vi "IV_Reader.vi"(6 "Sweep parameters":T1={"Vbg"=15.0, "Vbg step"=0.0, "Vsg"=-0.5, "Vsg step"=0.025, "B"=0.0, "B step"=0.0, "Temp"=2.0, "Temp step"=0.0}, 7 "Path to PNG Folder":path=path "C:/Users/ansom/Desktop/Agilent/PNG's From Graphs/B_BG_7to-7", 8 "Use only a subset of the folder":bool, 9 "Subset Length":i32=41, 10 "Subset Index":i32=2624, 11 "Folder or File":path=path "D:/SA03008H.20180718/77_B+SG_B_-7to0inc1_SG_-0.5to0.5inc0.25_at0.2Hz_-300mVto-100mV_IV_@BG15") -> (3 "dIdV_Intensity_Output":dbl[][](array[numeric]))   [LabVIEW 2016]
uses:
  <userlib>/LevyLab/LV to ITX/LVtoITX.lvclass
  <vilib>/Analysis/NI_AALBase.lvlib
  <vilib>/MakerHub/Toolbox/LMH-Toolbox.lvlib
  <vilib>/Analysis/1siggen.llb/Ramp Pattern by Delta.vi
panel:
  out "initialized array":dbl[](array[numeric])
  out "output array":dbl[](array[numeric])
  out "output cluster":cluster{dbl[], dbl[], dbl[]}
  in  "Sgstep":dbl
  in  "Sgstart":dbl
  in  "T-Slider, F-AutoChopper":bool
  in  "dI/dV OFFSET":dbl=100.0 format="%#_13g"
  in  "IV OFFSET":dbl format="%#_13g"
  in  "e^2/h ?":bool
  in  "X step":dbl
  in  "X start":dbl
  out "Differential Conductance":dbl[][](graph)
  in  "Portion of data":cluster{dbl, dbl}(slide)={1.0, 0.0} scale=0.0..1.0
  out "Iterations of loop":i32=40
  out "directory":bool=TRUE
  out "dI/dV":cluster{dbl[], dbl[]}[](graph)
  out "A vs B":cluster{dbl[], dbl[]}[](graph)
  in  "Diff bin size":dbl
  out "Comments":string="IGOR\nX// Date: 7/19/2018 8:23 PM\nX// SA03008H\nX// \nX// Trying to see what the stepping stuff looks like up close\nX// \nX// Source 2 Drain 28 (lockin 1 and 7)\nX// Gohm resistor, sweep SG\nX// \nX// 100mV AC -200mV DC for the IV sweep\nX// \nX// -0.5 to 0.5 @ 0.025 V step sizes\nX// B at 4T now\n\nX// DSA_Vsg1=0.500000\n\nX// \nX// B= 3.999994\n\n\n\n\n\n\n\n\n\n\n\n\n\n\n\n\n\n\n\n\n\n\n\n\n\n\n\n\n\n\n\n\n\n\n\n\n\n\n\n\nX \nX Display/R 'time.SA03008H.20180718.000040'\nX AppendToGraph 'temp.SA03008H.20180718.000040'\nX AppendToGraph 'B.SA03008H.20180718.000040'\nX AppendToGraph 'Vsource.SA03008H.20180718.000040'\nX AppendToGraph 'Lockin0.SA03008H.20180718.000040'\nX AppendToGraph 'Lockin1.SA03008H.20180718.000040'\nX AppendToGraph 'Lockin2.SA03008H.20180718.000040'\nX AppendToGraph 'Lockin3.SA03008H.20180718.000040'\nX AppendToGraph 'Lockin4.SA03008H.20180718.000040'\nX AppendToGraph 'Lockin5.SA03008H.20180718.000040'\nX AppendToGraph 'B_rate.SA03008H.20180718.000040'\nX AppendToGraph 'DC0.SA03008H.20180718.000040'\nX AppendToGraph 'DC1.SA03008H.20180718.000040'\nX AppendToGraph 'DC2.SA03008H.20180718.000040'\nX AppendToGraph 'DC3.SA03008H.20180718.000040'\nX AppendToGraph 'DC4.SA03008H.20180718.000040'\nX AppendToGraph 'DC5.SA03008H.20180718.000040'\nX AppendToGraph 'DC6.SA03008H.20180718.000040'\nX AppendToGraph 'DC7.SA03008H.20180718.000040'\nX Label bottom \"x label\"\nX Label left \"y label\"\nX ModifyGraph rgb('time.SA03008H.20180718.000040')=(65280,0,0)\nX ModifyGraph rgb('temp.SA03008H.20180718.000040')=(65280,18432,0)\nX ModifyGraph rgb('B.SA03008H.20180718.000040')=(65280,36864,0)\nX ModifyGraph rgb('Vsource.SA03008H.20180718.000040')=(65280,55296,0)\nX ModifyGraph rgb('Lockin0.SA03008H.20180718.000040')=(57344,65280,0)\nX ModifyGraph rgb('Lockin1.SA03008H.20180718.000040')=(37376,65280,0)\nX ModifyGraph rgb('Lockin2.SA03008H.20180718.000040')=(18944,65280,0)\nX ModifyGraph rgb('Lockin3.SA03008H.20180718.000040')=(512,65280,0)\nX ModifyGraph rgb('Lockin4.SA03008H.20180718.000040')=(0,65280,17920)\nX ModifyGraph rgb('Lockin5.SA03008H.20180718.000040')=(0,65280,36352)\nX ModifyGraph rgb('B_rate.SA03008H.20180718.000040')=(0,65280,54784)\nX ModifyGraph rgb('DC0.SA03008H.20180718.000040')=(0,57856,65280)\nX ModifyGraph rgb('DC1.SA03008H.20180718.000040')=(0,39424,65280)\nX ModifyGraph rgb('DC2.SA03008H.20180718.000040')=(0,20992,65280)\nX ModifyGraph rgb('DC3.SA03008H.20180718.000040')=(0,2560,65280)\nX ModifyGraph rgb('DC4.SA03008H.20180718.000040')=(17408,0,65280)\nX ModifyGraph rgb('DC5.SA03008H.20180718.000040')=(35840,0,65280)\nX ModifyGraph rgb('DC6.SA03008H.20180718.000040')=(54272,0,65280)\nX ModifyGraph rgb('DC7.SA03008H.20180718.000040')=(65280,0,58368)\nX Legend/C/N=text0/J \"\\\\s('time.SA03008H.20180718.000040') time\\r\\\\s('temp.SA03008H.20180718.000040') temp\\r\\\\s('B.SA03008H.20180718.000040') B\\r\\\\s('Vsource.SA03008H.20180718.000040') Vsource\\r\\\\s('Lockin0.SA03008H.20180718.000040') Lockin0\\r\\\\s('Lockin1.SA03008H.20180718.000040') Lockin1\\r\\\\s('Lockin2.SA03008H.20180718.000040') Lockin2\\r\\\\s('Lockin3.SA03008H.20180718.000040') Lockin3\\r\\\\s('Lockin4.SA03008H.20180718.000040') Lockin4\\r\\\\s('Lockin5.SA03008H.20180718.000040') Lockin5\\r\\\\s('B_rate.SA03008H.20180718.000040') B_rate\\r\\\\s('DC0.SA03008H.20180718.000040') DC0\\r\\\\s('DC1.SA03008H.20180718.000040') DC1\\r\\\\s('DC2.SA03008H.20180718.000040') DC2\\r\\\\s('DC3.SA03008H.20180718.000040') DC3\\r\\\\s('DC4.SA03008H.20180718.000040') DC4\\r\\\\s('DC5.SA03008H.20180718.000040') DC5\\r\\\\s('DC6.SA03008H.20180718.000040') DC6\\r\\\\s('DC7.SA03008H.20180718.000040') DC7\"\nX ModifyGraph mirror(bottom)=1\nX ModifyGraph width=216\nX ModifyGraph height={Aspect,0.6}\nX ModifyGraph Log(bottom)=0\nX ModifyGraph Log(left)=0\nX \n"
  in  "Diff bin size":dbl=2.0
  out "N__":cluster{"N1":dbl, "N2":dbl, "N3":dbl, "N4":dbl}={"N1"=3614891004.465372, "N2"=3614891004.465372, "N3"=3614891004.465372, "N4"=3614891004.465372} {"N4" format="%#_6p"; "N3" format="%#_6p"; "N2" format="%#_6p"; "N1" format="%#_6p"}
  out "IV":dbl[][](graph)
  in  "index":T2={"A"=5, "B"=3, "C"=2, "D"=0, "E"=3, "N1"=0, "N2"=0, "N3"=0, "N4"=0}
  # "YES"
  # "NO"
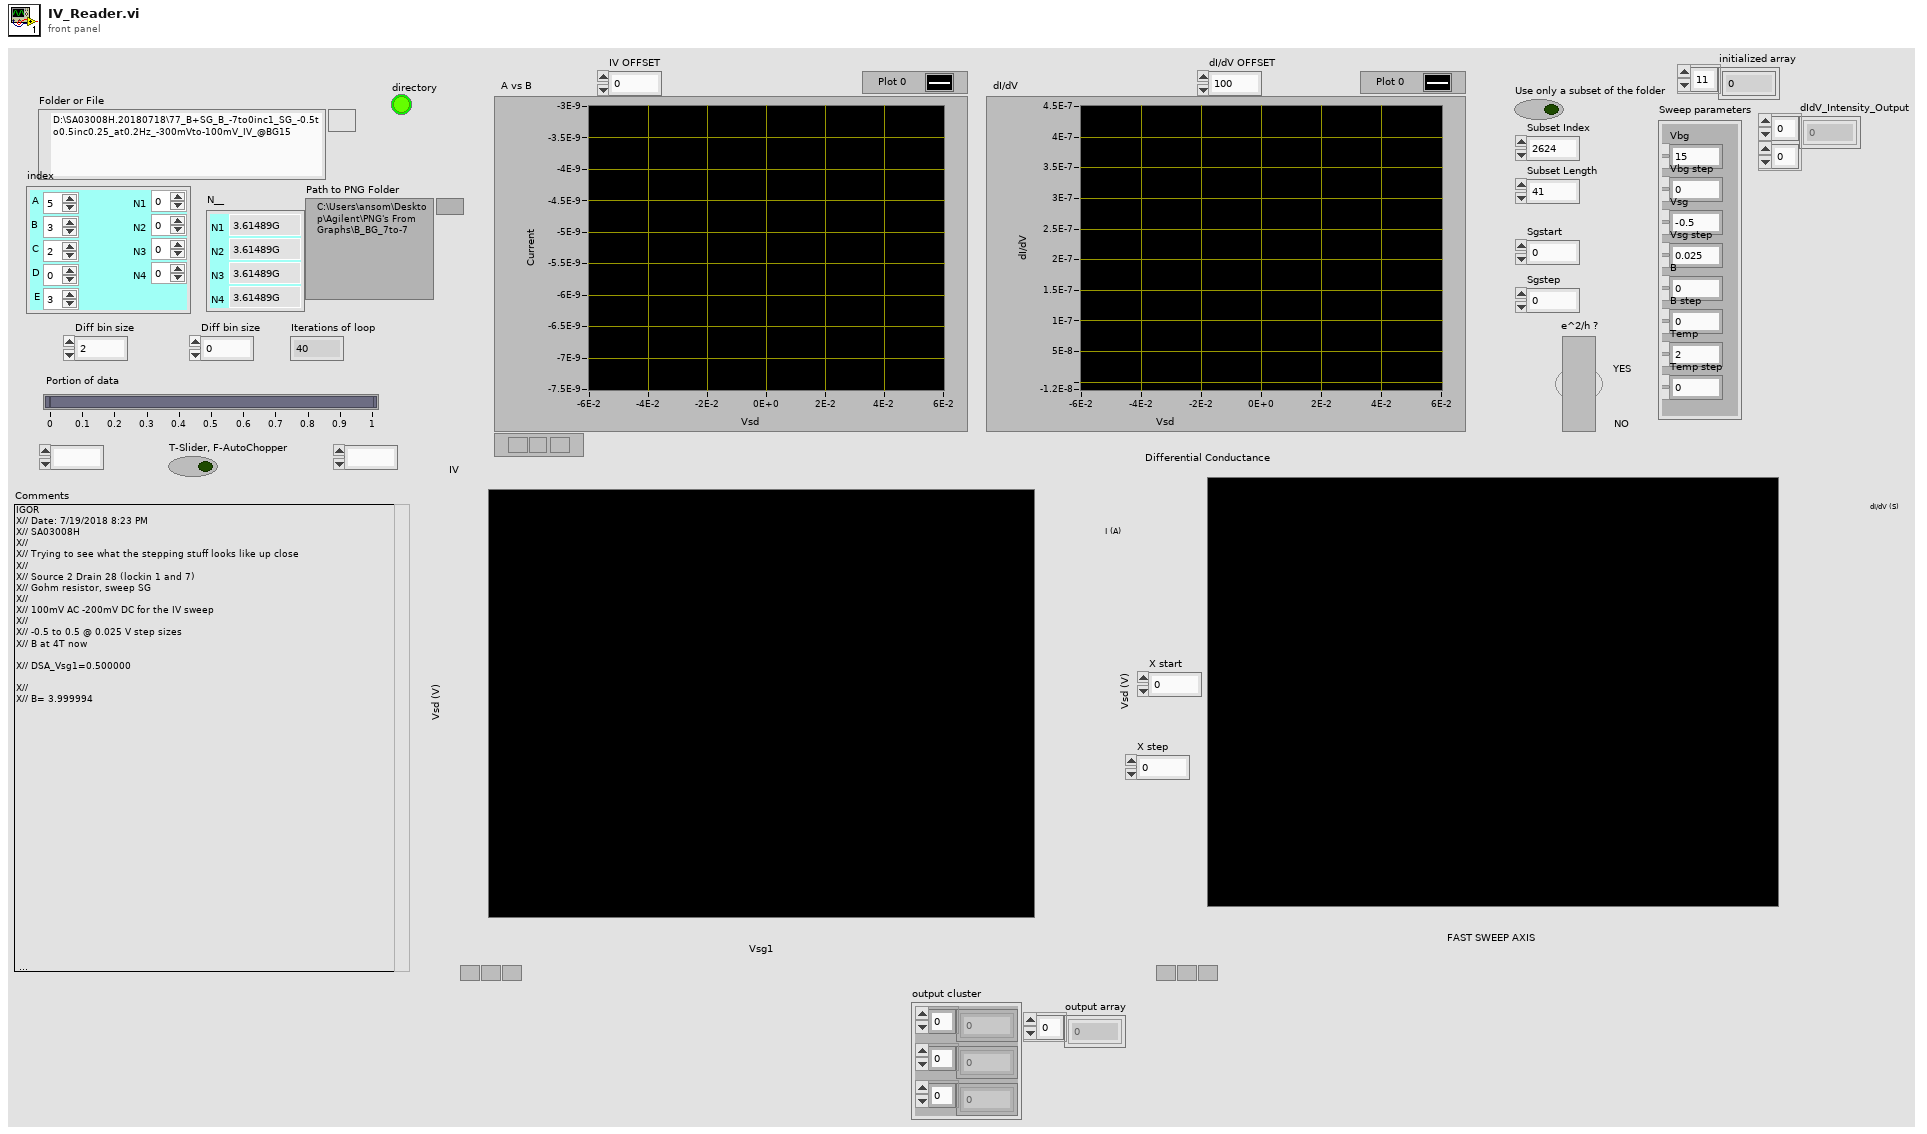
[diagram p1: front panel]
types:
  T1 = cluster{"Vbg":dbl, "Vbg step":dbl, "Vsg":dbl, "Vsg step":dbl, "B":dbl, "B step":dbl, "Temp":dbl, "Temp step":dbl}
  T2 = cluster{"A":i32, "B":i32, "C":i32, "D":i32, "E":i32, "N1":i32, "N2":i32, "N3":i32, "N4":i32}
  T3 = cluster{"Decimated Array":dbl[], "Decimated Array":dbl[]}[]
  T4 = cluster{"Decimated Array":dbl[], "Decimated Array":dbl[]}
  T5 = typedef "imagedata.ctl" = cluster{"image type":i32, "image depth":i32, "image":u8[], "mask":u8[], "colors":u32[], "Rectangle":cluster{"left":i16, "top":i16, "right":i16, "bottom":i16}}
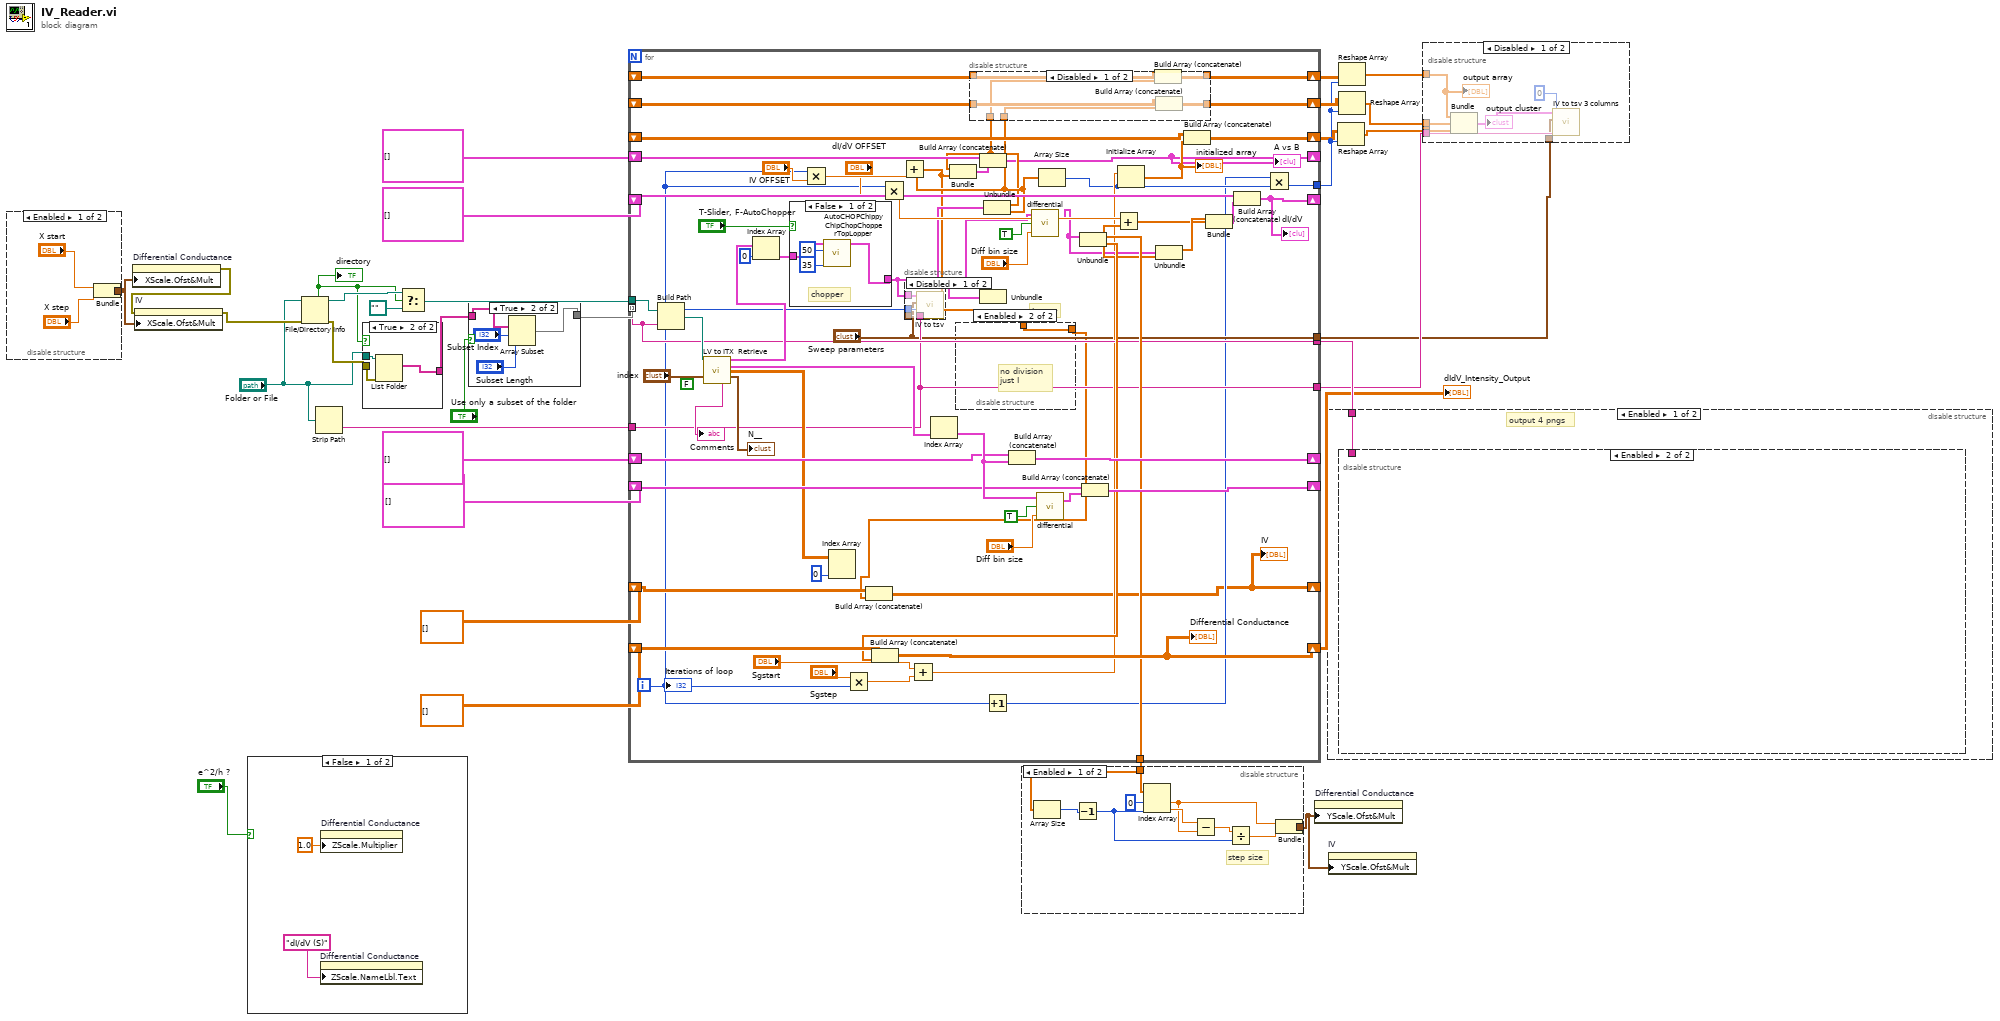
[diagram p0: block diagram]
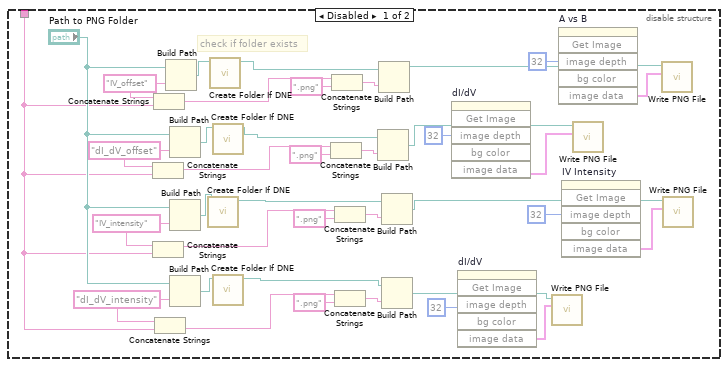
[diagram p3: hidden frame]
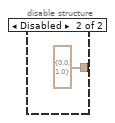
[diagram p6: hidden frame]
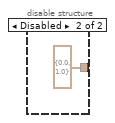
[diagram p7: hidden frame]
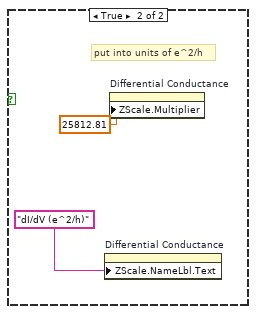
[diagram p8: hidden frame]
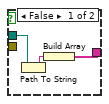
[diagram p9: hidden frame]
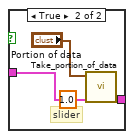
[diagram p12: hidden frame]
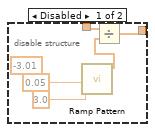
[diagram p13: hidden frame]
diagram:
  n1 = disable-structure shown="Enabled" {
    disable-tunnel: [w34 cluster{"X start":dbl, "X step":dbl} {"X start"=0.0, "X step"=1.0}] -> w21
    frame Enabled {
      n2 = Bundle("X start"="X start", "X step"="X step") -> (w34:cluster{"X start":dbl, "X step":dbl})  [unwired: 1 in]
    }
    frame Disabled {
    }
  }
  n3 = property on="Differential Conductance" class="IntGraph (strict)"("XScale.Ofst&Mult"=w21) -> (error out=w19:errorcluster)  [unwired: 2 in, 1 out]
  n4 = property on="IV" class="IntGraph (strict)"(error in=w19, "XScale.Ofst&Mult"=w21) -> (error out=w18:errorcluster)  [unwired: 1 in, 1 out]
  n5 = case shown="False" "e^2/h ?" {
    frame False {
      n6 = property on="Differential Conductance" class="IntGraph (strict)"("ZScale.Multiplier"=1.0 ("Z Scale.Offset and Multiplier:Multiplier")) -> ()  [unwired: 2 in, 2 out]
      n7 = property on="Differential Conductance" class="IntGraph (strict)"("ZScale.NameLbl.Text"="dI/dV (S)" ("Z Scale.Unit Label.Text")) -> ()  [unwired: 2 in, 2 out]
    }
    frame True {
      # "put into units of e^2/h"
      n8 = property on="Differential Conductance" class="IntGraph (strict)"("ZScale.NameLbl.Text"="dI/dV (e^2/h)" ("Z Scale.Unit Label.Text")) -> ()  [unwired: 2 in, 2 out]
      n9 = property on="Differential Conductance" class="IntGraph (strict)"("ZScale.Multiplier"=25812.81 ("Z Scale.Offset and Multiplier:Multiplier")) -> ()  [unwired: 2 in, 2 out]
    }
  }
  n10 = File/Directory Info(path="Folder or File", error in=w18) -> (path out=w27:path, directory=w26:bool, error out=w28:errorcluster)  [unwired: 4 out]
  "directory" <- w26
  n11 = Strip Path(path="Folder or File") -> (name=w11:string)  [unwired: 1 out]
  n12 = case shown="True" w26 {
    tunnel: "Folder or File" -> [w44 w47]
    tunnel: w28 -> [_ w46]
    tunnel: [w42 w45] -> w15
    frame False {
      n13 = Path To String(path=w44) -> (string=w43:string)
      n14 = Build Array(w43) -> (w42:string[])
    }
    frame True {
      n15 = List Folder(path=w47, error in=w46) -> (filenames=w45:string[])  [unwired: 2 in, 3 out]
    }
  }
  n16 = Select(t=w27, s=w26, f=path "") -> (s? t:f=w25:path)
  n17 = case shown="True" "Use only a subset of the folder" {
    tunnel: w15 -> [w48 w52]
    tunnel: [w48 w51] -> w14
    frame False {
    }
    frame True {
      n18 = Array Subset(array=w52, index="Subset Index", length="Subset Length") -> (w51:string[])
    }
  }
  n19 = for {
    shift-right: [w54] -> _
    shift-left: cluster{dbl[], dbl[]}[] [] -> [w112]
    shift-right: [w55] -> _
    shift-left: T3 [] -> [w111]
    shift-right: [w102] -> _
    shift-left: T3 [] -> [w106]
    shift-right: [w103] -> _
    shift-left: cluster{dbl[], dbl[]}[] [] -> [w105]
    tunnel: w14 -> [w77] mode=indexing
    shift-right: [w53] -> _
    shift-left: dbl[][] [] -> [w99]
    tunnel: w25 -> [w98]
    shift-right: [w94] -> w1
    shift-left: dbl[][] [] -> [w96]
    tunnel: [w93] -> w22
    tunnel: [w77] -> w16
    tunnel: w11 -> [w64]
    shift-right: [w71] -> w10
    shift-left: _ -> [w70]
    shift-right: [w68] -> w9
    shift-left: _ -> [w67]
    shift-right: [w66] -> w8
    shift-left: _ -> [w65]
    tunnel: [w64] -> w4
    tunnel: ["Sweep parameters"] -> w3
    tunnel: [w61] -> w2
    i -> [w60]
    (unwired) FALSE ("stop")
    # "I array"
    n20 = Build Path(base path=w98, name or relative path=w77) -> (appended path=w104:path)
    n21 = call <userlib>:"LV to ITX  Retrieve.vi"("File or Folder Path"=w104, "index"="index") -> ("A vs B"=w81:cluster{dbl[], dbl[]}[], "C vs D"=w97:cluster{dbl[], dbl[]}[], "E"=w101:dbl[][], "N"=→"N__":cluster{"N1":dbl, "N2":dbl, "N3":dbl, "N4":dbl}, "Comments"=→"Comments":string)  [unwired: 9 in]
    n22 = Index Array(array=w81, index=0) -> (element=w80:cluster{dbl[], dbl[]})
    n23 = case shown="False" "T-Slider, F-AutoChopper" {
      tunnel: [w128 w133] -> w78
      tunnel: w80 -> [w131 w132]
      frame False {
        # "chopper"
        n24 = call "AutoCHOPChippyChipChopChopperTopLopper.vi"("Points to chop off the bottom edge"=35, "Points to chop off the top edge"=50, "Vsrc and Current In"=w131) -> ("Vsrc and Current Out"=w128:cluster{dbl[], dbl[]})  [unwired: 8 in]
      }
      frame True {
        (unwired) 1.0 ("Decimate point")
        # "slider"
        n25 = call <userlib>:"Take_portion_of_data.vi"("input IV"=w132, "Slide"="Portion of data") -> ("Output IV"=w133:cluster{dbl[], dbl[]})  [unwired: 5 in]
      }
    }
    n26 = Multiply(x=w60, y="IV OFFSET") -> (x*y=w90:dbl)
    n27 = Index Array(array=w101, index (col)=0 ("index (row)")) -> ()  [unwired: 1 in, 1 out]
    n28 = Multiply(x="Sgstep", y=w60) -> (x*y=w74:dbl)
    n29 = Multiply(x=w60, y="dI/dV OFFSET") -> (x*y=w89:dbl)
    n30 = disable-structure shown="Disabled" {
      disable-tunnel: w78 -> [w127 _]
      disable-tunnel: w60 -> [w126 _]
      disable-tunnel: "Sweep parameters" -> [w125 _]
      disable-tunnel: w64 -> [w124 _]
      frame Disabled {
        n31 = call "IV to tsv.vi"("experiment name"=w124, "Iteration"=w126, "Sweep parameters"=w125, "Output IV"=w127) -> ()  [unwired: 8 in]
      }
      frame Enabled {
      }
    }
    n32 = Add(x="Sgstart", y=w74) -> (x+y=w73:dbl)
    n33 = Index Array(array=w97) -> (element=w109:cluster{dbl[], dbl[]})  [unwired: 1 in]
    n34 = Unbundle(w78) -> ()  [unwired: 2 out]
    n35 = Unbundle(w78) -> (w58:dbl[], w69:dbl[])
    n36 = Add(x=w90, y=w69) -> (x+y=w57:dbl[])
    n37 = Bundle(w58, w57) -> (w91:cluster{dbl[], dbl[]})  [unwired: 1 in]
    n38 = disable-structure shown="Enabled" {
      disable-tunnel: w57 -> [w137 w141]
      disable-tunnel: [w135 w141] -> w56
      frame Disabled {
        n39 = call-poly <vilib>:"Ramp Pattern.vi"("start"=-3.01, "end"=3.0, "delta"=0.05) -> ("Ramp Pattern"=w136:dbl[])  [unwired: 6 in, 2 out]
        n40 = Divide(x=w137, y=w136) -> (x/y=w135:dbl[])
      }
      frame Enabled {
        # "no division\njust I"
      }
    }
    n41 = Build Array (concatenate)(w99, w56) -> (w53:dbl[][])
    "IV" <- w53
    n42 = disable-structure shown="Disabled" {
      disable-tunnel: w69 -> [w123 _]
      disable-tunnel: [w122 _] -> w68
      disable-tunnel: w67 -> [w121 _]
      disable-tunnel: [w120 _] -> w66
      disable-tunnel: w65 -> [w119 _]
      disable-tunnel: w58 -> [w118 _]
      frame Disabled {
        n43 = Build Array (concatenate)(w119, w118) -> (w120:dbl[][])
        n44 = Build Array (concatenate)(w121, w123) -> (w122:dbl[][])
      }
      frame Enabled {
      }
    }
    n45 = Build Array (concatenate)(w112, w91) -> (w54:cluster{dbl[], dbl[]}[])
    "A vs B" <- w54
    n46 = Increment(x=w60) -> (x+1=w59:i32)
    n47 = Build Array (concatenate)(w105, w109) -> (w103:cluster{dbl[], dbl[]}[])
    n48 = call <userlib>:"differential.vi"("Numeric"="Diff bin size", "dy/dx vs x"=TRUE, "A vs B 2"=w78) -> ("A vs B 3"=w84:T4)  [unwired: 1 in]
    n49 = call <userlib>:"differential.vi"("Numeric"="Diff bin size", "dy/dx vs x"=TRUE, "A vs B 2"=w109) -> ("A vs B 3"=w110:T4)  [unwired: 1 in]
    n50 = Array Size(array=w69) -> (size(s)=w62:i32)
    n51 = Unbundle(w84) -> ("Decimated Array"=w93:dbl[], "Decimated Array"=w95:dbl[])
    n52 = Build Array (concatenate)(w96, w95) -> (w94:dbl[][])
    "Differential Conductance" <- w94
    n53 = Build Array (concatenate)(w106, w110) -> (w102:T3)
    n54 = Initialize Array(w73, w62) -> (w72:dbl[])
    "initialized array" <- w72
    n55 = Unbundle(w84) -> ("Decimated Array"=w86:dbl[], "Decimated Array"=w87:dbl[])
    n56 = Add(x=w89, y=w87) -> (x+y=w83:dbl[])
    n57 = Build Array (concatenate)(w70, w72) -> (w71:dbl[][])
    n58 = Bundle("Decimated Array"=w86, w83) -> (w85:cluster{"Decimated Array":dbl[], dbl[]})  [unwired: 1 in]
    n59 = Build Array (concatenate)(w111, w85) -> (w55:T3)
    "dI/dV" <- w55
    n60 = Multiply(x=w59, y=w62) -> (x*y=w61:i32)
    "Iterations of loop" <- w60
  }
  "dIdV_Intensity_Output" <- w1
  n61 = disable-structure shown="Enabled" {
    disable-tunnel: w22 -> [w149 _]
    disable-tunnel: [w142 cluster{dbl, dbl} {0.0, 1.0}] -> w20
    frame Enabled {
      # "step size"
      n62 = Array Size(array=w149) -> (size(s)=w146:i32)
      n63 = Decrement(x=w146) -> (x-1=w145:i32)
      n64 = Index Array(array=w149, index #1=0 ("index"), index #2=w145) -> (element #1=w144:dbl, element #2=w148:dbl)
      n65 = Subtract(x=w148, y=w144) -> (x-y=w147:dbl)
      n66 = Divide(x=w147, y=w145) -> (x/y=w143:dbl)
      n67 = Bundle(w144, w143) -> (w142:cluster{dbl, dbl})  [unwired: 1 in]
    }
    frame Disabled {
    }
  }
  n68 = property on="Differential Conductance" class="IntGraph (strict)"("YScale.Ofst&Mult"=w20) -> ()  [unwired: 2 in, 2 out]
  n69 = disable-structure shown="Enabled" {
    disable-tunnel: w16 -> [w152 _]
    frame Enabled {
      # "output 4 pngs"
      n70 = disable-structure shown="Enabled" {
        disable-tunnel: w152 -> [w183 _]
        frame Disabled {
          w184 = "dI_dV_intensity" ("name or relative path")
          w185 = "IV_intensity" ("name or relative path")
          w186 = "dI_dV_offset" ("name or relative path")
          w187 = "IV_offset" ("name or relative path")
          # "check if folder exists"
          n71 = Concatenate Strings(w186, w183) -> (w173:string)
          n72 = Concatenate Strings(w185, w183) -> (w174:string)
          n73 = Concatenate Strings(w187, w183) -> (w182:string)
          n74 = Concatenate Strings(w184, w183) -> (w175:string)
          n75 = Build Path(base path="Path to PNG Folder", name or relative path=w187) -> (appended path=w160:path)
          n76 = Build Path(base path="Path to PNG Folder", name or relative path=w186) -> (appended path=w153:path)
          n77 = Build Path(base path="Path to PNG Folder", name or relative path=w185) -> (appended path=w156:path)
          n78 = Build Path(base path="Path to PNG Folder", name or relative path=w184) -> (appended path=w158:path)
          n79 = call <vilib>:"Create Folder If DNE.vi"("Folder Path"=w156) -> ("Dup Path"=w155:path)  [unwired: 9 in, 1 out]
          n80 = call <vilib>:"Create Folder If DNE.vi"("Folder Path"=w160) -> ("Dup Path"=w159:path)  [unwired: 9 in, 1 out]
          n81 = call <vilib>:"Create Folder If DNE.vi"("Folder Path"=w153) -> ("Dup Path"=w154:path)  [unwired: 9 in, 1 out]
          n82 = call <vilib>:"Create Folder If DNE.vi"("Folder Path"=w158) -> ("Dup Path"=w157:path)  [unwired: 9 in, 1 out]
          n83 = Concatenate Strings(w173, ".png" ("string")) -> (w180:string)
          n84 = Concatenate Strings(w182, ".png" ("string")) -> (w190:string)
          n85 = Concatenate Strings(w174, ".png" ("string")) -> (w179:string)
          n86 = Concatenate Strings(w175, ".png" ("string")) -> (w176:string)
          n87 = Build Path(base path=w154, name or relative path=w180) -> (appended path=w164:path)
          n88 = Build Path(base path=w159, name or relative path=w190) -> (appended path=w172:path)
          n89 = Build Path(base path=w155, name or relative path=w179) -> (appended path=w168:path)
          n90 = Build Path(base path=w157, name or relative path=w176) -> (appended path=w161:path)
          n91 = invoke on="dI/dV" class="XYGraph (strict)" method="Get Image"("image depth"=32 ("Image Depth")) -> ("image data"=w165:T5)  [unwired: 5 in, 5 out]
          n92 = invoke on="dI/dV" class="IntGraph (strict)" method="Get Image"("image depth"=32 ("Image Depth")) -> ("image data"=w162:T5)  [unwired: 5 in, 5 out]
          n93 = call <vilib>:"Write PNG File.vi"("image data"=w162, "path to PNG file"=w161) -> ()  [unwired: 8 in, 2 out]
          n94 = invoke on="A vs B" class="XYGraph (strict)" method="Get Image"("image depth"=32 ("Image Depth")) -> ("image data"=w170:T5)  [unwired: 5 in, 5 out]
          n95 = invoke on="IV Intensity" class="IntGraph (strict)" method="Get Image"("image depth"=32 ("Image Depth")) -> ("image data"=w169:T5)  [unwired: 5 in, 5 out]
          n96 = call <vilib>:"Write PNG File.vi"("image data"=w165, "path to PNG file"=w164) -> ()  [unwired: 8 in, 2 out]
          n97 = call <vilib>:"Write PNG File.vi"("image data"=w170, "path to PNG file"=w172) -> ()  [unwired: 8 in, 2 out]
          n98 = call <vilib>:"Write PNG File.vi"("image data"=w169, "path to PNG file"=w168) -> ()  [unwired: 8 in, 2 out]
        }
        frame Enabled {
        }
      }
    }
    frame Disabled {
    }
  }
  n99 = property on="IV" class="IntGraph (strict)"("YScale.Ofst&Mult"=w20) -> ()  [unwired: 2 in, 2 out]
  n100 = Reshape Array(w10, w2) -> (w5:dbl[])
  n101 = Reshape Array(w8, w2) -> (w7:dbl[])
  n102 = Reshape Array(w9, w2) -> (w6:dbl[])
  n103 = disable-structure shown="Disabled" {
    disable-tunnel: w7 -> [w197 _]
    disable-tunnel: w6 -> [w196 _]
    disable-tunnel: w5 -> [w195 _]
    disable-tunnel: w4 -> [w193 _]
    disable-tunnel: w3 -> [w192 _]
    frame Disabled {
      n104 = Bundle(w197, w196, w195) -> (w194:cluster{dbl[], dbl[], dbl[]})  [unwired: 1 in]
      "output cluster" <- w194
      n105 = call "IV to tsv 3 columns.vi"("experiment name"=w193, "Iteration"=0, "Sweep parameters"=w192, "output cluster"=w194) -> ()  [unwired: 8 in]
      "output array" <- w197
    }
    frame Enabled {
    }
  }
